vi "Add Config Section.vi"(8 "error in (no error)":errorcluster, 10 "FileName":string, 11 "Editor.lvclass in":refnum<data-value>) -> (0 "error out":errorcluster, 3 "Editor.lvclass out":refnum<data-value>)   [LabVIEW 2015, in "Editor.lvclass"]
uses:
  Editor.lvclass
  Project.lvclass
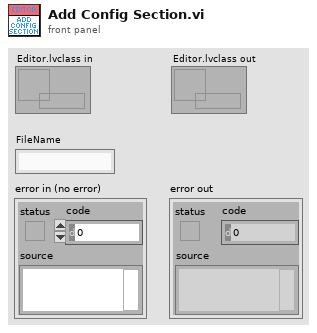
[diagram p1: front panel]
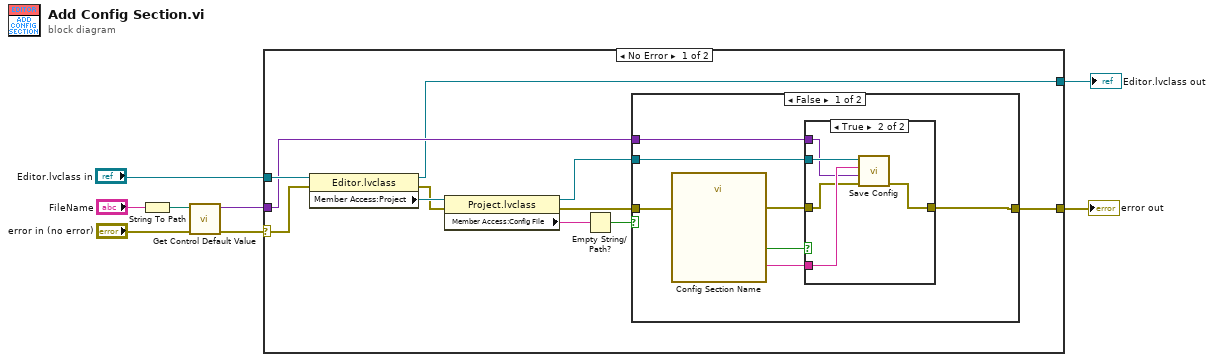
[diagram p0: block diagram]
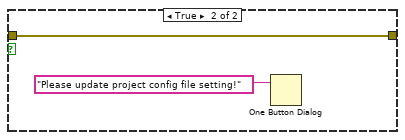
[diagram p3: hidden frame]
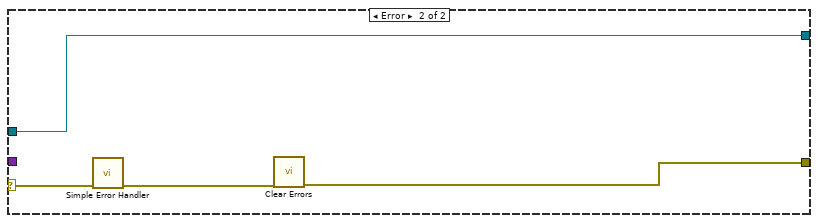
[diagram p4: hidden frame]
diagram:
  n1 = String To Path(string="FileName") -> (path=w7:path)
  n2 = call "Get Control Default Value.vi"("error in (no error)"="error in (no error)", "Path"=w7) -> ("error out"=w5:errorcluster, "Value"=w4:variant)  [unwired: 8 in]
  n3 = case shown="No Error" w5 {
    selector: w5 -> [w17 w38]
    tunnel: w4 -> [w13 _]
    tunnel: "Editor.lvclass in" -> [w19 w35]
    tunnel: [w10 w36] -> w3
    tunnel: [w11 w35] -> w1
    frame No Error {
      n4 = property class="Editor.lvclass"(reference=w19, error in=w17) -> (reference out=w11:refnum<data-value>, error out=w16:errorcluster, "Member Access:Project"=w18:refnum<class "Project.lvclass">)
      n5 = property class="Project.lvclass"(reference=w18, error in=w16) -> (reference out=w9:refnum<class "Project.lvclass">, error out=w12:errorcluster, "Member Access:Config File"=w14:string)
      n6 = Empty String/Path?(string/path=w14) -> (empty?=w15:bool)
      n7 = case shown="False" w15 {
        tunnel: w13 -> [w26 _]
        tunnel: w12 -> [w23 w33]
        tunnel: [w21 w33] -> w10
        tunnel: w9 -> [w20 _]
        frame False {
          n8 = call "Config Section Name"("error in (no error)"=w23) -> ("Section Name"=w24:string, "OK"=w25:bool, "error out"=w22:errorcluster)  [unwired: 16 in]
          n9 = case shown="True" w25 {
            tunnel: w26 -> [_ w30]
            tunnel: w24 -> [_ w31]
            tunnel: w22 -> [w27 w29]
            tunnel: [w27 w28] -> w21
            tunnel: w20 -> [_ w32]
            frame False {
            }
            frame True {
              n10 = call "Save Config.vi"("error in (no error)"=w29, "Value in"=w30, "Section"=w31, "Project in"=w32) -> ("error out"=w28:errorcluster)  [unwired: 6 in, 1 out]
            }
          }
        }
        frame True {
          n11 = One Button Dialog(message="Please update project config file setting!") -> ()  [unwired: 1 in, 1 out]
        }
      }
    }
    frame Error {
      n12 = call <vilib>:"Simple Error Handler.vi"("error in (no error)"=w38) -> ("error out"=w37:errorcluster)  [unwired: 4 in, 4 out]
      n13 = call <vilib>:"Clear Errors.vi"("error in (no error)"=w37) -> ("error out"=w36:errorcluster)  [unwired: 5 in, 1 out]
    }
  }
  "error out" <- w3
  "Editor.lvclass out" <- w1
